vi "AB_Log_SaveClose_Source_Item.vi"(6 "index":i32, 7 "initial time":u32, 8 "error in (no error)":errorcluster, 9 "saveLevel":u32, 10 "destinationPath":path, 11 "sourcePath":path) -> (0 "error out":errorcluster)   [LabVIEW 2020]
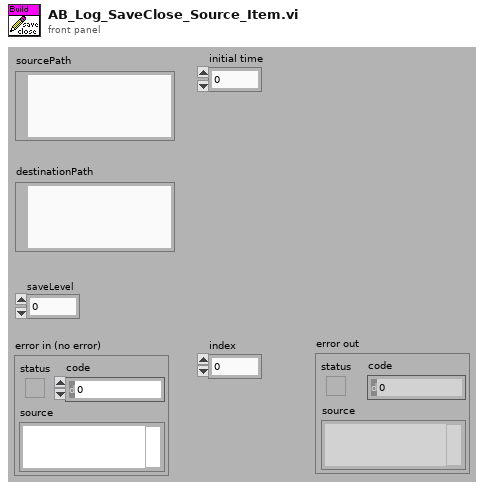
[diagram p1: front panel]
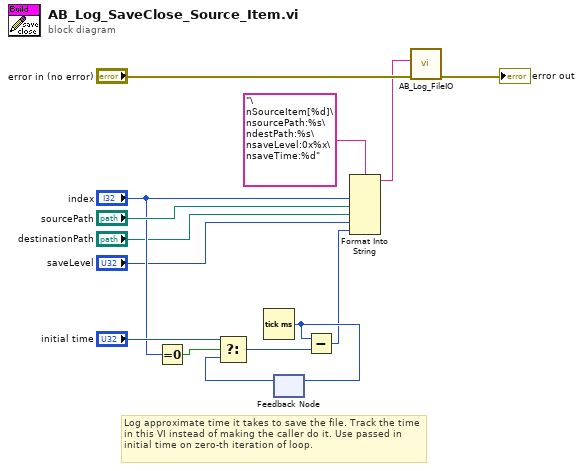
[diagram p0: block diagram]
diagram:
  # "Log approximate time it takes to save the file. Track the time in this VI instead of making the caller do it. Use passed in initial time on zero-th iteration of loop."
  n1 = Equal To 0?(x="index") -> (x = 0?=w9:bool)
  n2 = Tick Count (ms)() -> (millisecond timer value=w8:u32)
  n3 = feedback-in #1(w8) -> ()
  n4 = feedback #1() -> (w7:u32)  [unwired: 1 out]
  n5 = Select(t="initial time", s=w9, f=w7) -> (s? t:f=w4:u32)
  n6 = Subtract(x=w8, y=w4) -> (x-y=w2:u32)
  n7 = Format Into String(format string="\nSourceItem[%d]\nsourcePath:%s\ndestPath:%s\nsaveLevel:0x%x\nsaveTime:%d", "index", "sourcePath", "destinationPath", "saveLevel", w2) -> (resulting string=w5:string)  [unwired: 2 in, 1 out]
  n8 = call <vilib>:"AB_Log_FileIO.vi"("error in (no error)"="error in (no error)", "data"=w5) -> ("error out"=→"error out":errorcluster)  [unwired: 3 in, 6 out]
